vi "Altitude Only.vi"() -> ()   [LabVIEW 2012]
panel:
  in  "OK Button":bool
  out "Altitude":dbl=888888.0
  # "Current Effective Latitude in Meters"
  # "WARNING"
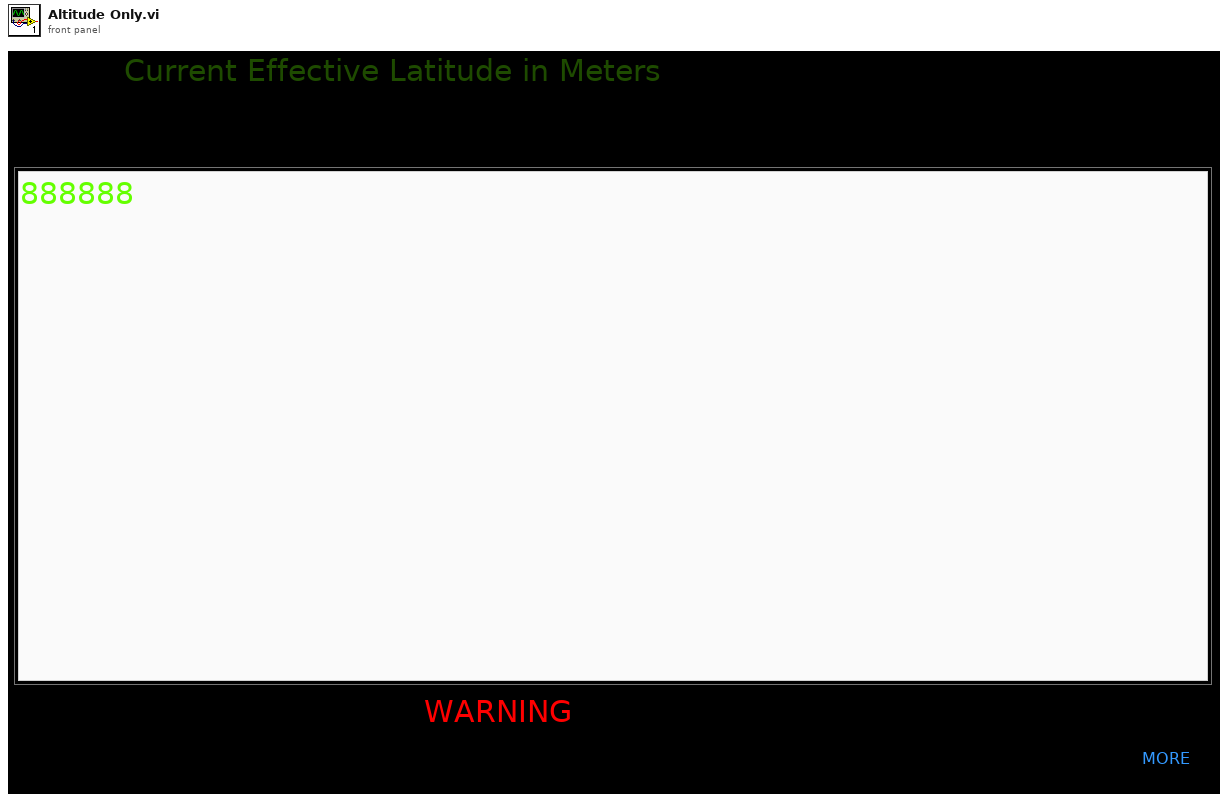
[diagram p1: front panel]
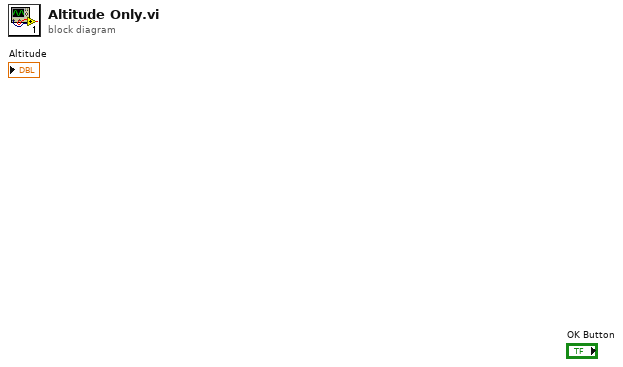
[diagram p0: block diagram]
diagram:
